vi "Node - PXImc Intial Handshaking.vi"(5 "Reader Buffer Size In":u64 caption="buffer size", 6 "Data In":u32[](array[numeric]), 7 "Connection Timeout (s)":dbl, 8 "error in (no error)":errorcluster, 9 "Reader Conn ID":u16=1 caption="writer's connection id (1)", 10 "Writer Conn ID":u16, 11 "Resource Name In":string) -> (0 "error out":errorcluster)   [LabVIEW 2016, in "PXImc Router.lvlib"]
uses:
  PXImc Router.lvlib
  <vilib>/pximc/Initialize Writer Session (U32).vi
  <vilib>/pximc/Initialize Reader Session (U32).vi
  <vilib>/pximc/Connect (U32).vi
  <vilib>/pximc/Write (U32).vi
  <vilib>/pximc/Read (U32).vi
  <vilib>/pximc/nipximc.lvlib
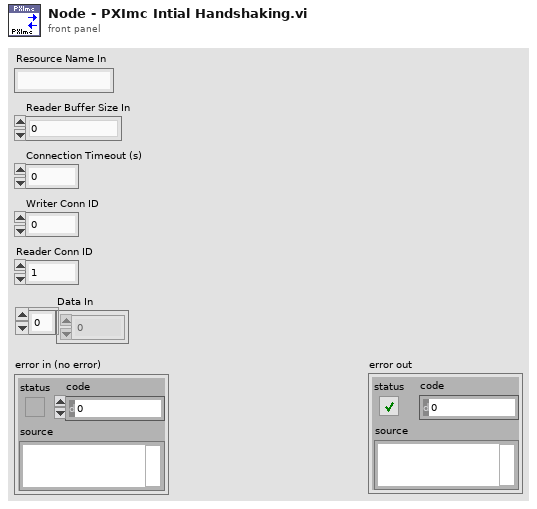
[diagram p1: front panel]
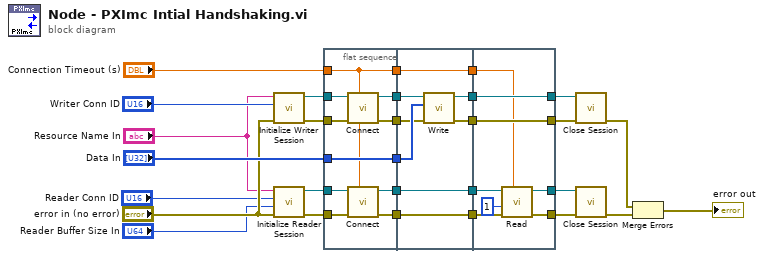
[diagram p0: block diagram]
diagram:
  n1 = call-poly <vilib>:"Initialize Writer Session.vi"("error in (no error)"="error in (no error)", "connection id (1)"="Writer Conn ID", "interface"="Resource Name In") -> ("error out"=w19:errorcluster, "session out"=w18:refnum<k21>)  [unwired: 7 in]
  n2 = call-poly <vilib>:"Initialize Reader Session.vi"("error in (no error)"="error in (no error)", "buffer size"="Reader Buffer Size In", "writer's connection id (1)"="Reader Conn ID", "interface"="Resource Name In") -> ("error out"=w17:errorcluster, "session out"=w15:refnum<k21>)  [unwired: 6 in]
  n3 = flat-sequence {
    tunnel: w18 -> [w39]
    tunnel: w19 -> [w38]
    tunnel: [w37] -> w26
    tunnel: [w36] -> w25
    tunnel: "Connection Timeout (s)" -> [w30]
    tunnel: "Data In" -> [w35]
    tunnel: [w35] -> w24
    tunnel: w17 -> [w34]
    tunnel: [w33] -> w16
    tunnel: w15 -> [w32]
    tunnel: [w31] -> w14
    tunnel: [w30] -> w5
    tunnel: w26 -> [w47]
    tunnel: w25 -> [w43]
    tunnel: [w46] -> w23
    tunnel: [w45] -> w22
    tunnel: w24 -> [w44]
    tunnel: w16 -> [w41]
    tunnel: w14 -> [w42]
    tunnel: [w42] -> w11
    tunnel: [w41] -> w10
    tunnel: w5 -> [w40]
    tunnel: [w40] -> w4
    tunnel: [w54] -> w21
    tunnel: [w55] -> w20
    tunnel: w23 -> [w55]
    tunnel: w22 -> [w54]
    tunnel: [w51] -> w12
    tunnel: [w50] -> w13
    tunnel: w11 -> [w53]
    tunnel: w10 -> [w52]
    tunnel: w4 -> [w48]
    frame #0 {
      n4 = call-poly <vilib>:"Connect.vi"("timeout in seconds (-1)"=w30, "error in (no error)"=w38, "session in"=w39) -> ("error out"=w36:errorcluster, "session out"=w37:refnum<k21>)  [unwired: 7 in]
      n5 = call-poly <vilib>:"Connect.vi"("timeout in seconds (-1)"=w30, "error in (no error)"=w34, "session in"=w32) -> ("error out"=w33:errorcluster, "session out"=w31:refnum<k21>)  [unwired: 7 in]
    }
    frame #1 {
      n6 = call-poly <vilib>:"Write.vi"("error in (no error)"=w43, "data"=w44, "session in"=w47) -> ("error out"=w45:errorcluster, "session out"=w46:refnum<k21>)  [unwired: 6 in, 1 out]
    }
    frame #2 {
      n7 = call-poly <vilib>:"Read.vi"("timeout in seconds (5)"=w48, "error in (no error)"=w52, "number of elements"=1, "session in"=w53) -> ("error out"=w51:errorcluster, "session out"=w50:refnum<k21>)  [unwired: 5 in, 1 out]
    }
  }
  n8 = call <vilib>:"Close Session.vi"("error in (no error)"=w21, "session in"=w20) -> ("error out"=w9:errorcluster)  [unwired: 9 in]
  n9 = call <vilib>:"Close Session.vi"("error in (no error)"=w12, "session in"=w13) -> ("error out"=w8:errorcluster)  [unwired: 9 in]
  n10 = Merge Errors(w9, w8) -> (→"error out":errorcluster)
